vi "Drive Teleop Handler.vi"(10 "Call Context":T1=enum."Stop") -> ()   [LabVIEW 2023]
uses:
  swerve/Type Definitions/Data/Robot Velocities.ctl
  <vilib>/Rock Robotics/WPI/DriverStation/WPI_DriverStationDerivedRobotMode.ctl
  Drive/Implementation/Driving Mode.ctl
  <vilib>/Rock Robotics/WPI/Joystick/XBox Buttons Indexer.ctl
  <vilib>/Rock Robotics/WPI/DriverStation/WPI_DriverStationAllianceInfo.ctl
  ce51abe2-3967-49ec-91df-d4b8ef358bb3.vi
  20f039dc-a6f5-4e97-88ba-31848a91c715.vi
  fdc21bd4-9215-41b8-8367-bf19dde4ba27.vi
  2558f998-dd4e-4154-8f44-6f70b21d0474.vi
  <vilib>/Rock Robotics/WPI/Utilities/WPI_GetSetVariantRefNum.vi
  <vilib>/Rock Robotics/Network Tables/NT Read Number.vi
  <vilib>/Rock Robotics/Network Tables/NT Read Boolean.vi
  Framework/Robot Global Data.vi
  <vilib>/Rock Robotics/Network Tables/NT Write Boolean.vi
panel:
  out "Astra Sees?":bool=TRUE
  out "Li4 Sees?":bool=TRUE
  in  "Red Side":cluster{"Upper lim":dbl, "Lower lim":dbl}={"Upper lim"=12.0, "Lower lim"=6.0}
  in  "Blue Side":cluster{"Upper lim":dbl, "Lower lim":dbl}={"Upper lim"=23.0, "Lower lim"=17.0}
  in  "Deadband Info":T2={"Deadband"=0.05, "Deadband High"=1.0, "Deadband Low"=0.05}
  in  "Max Velocities":T3={"X Velocity"=15.0, "Y Velocity"=15.0, "Rotational \nVelocity"=270.0}
  in  "Sinusoidal Terms":cluster{"Max Velocity":dbl, "Frequency":dbl}
  in  "Teleop Mode":T4(ring)
  in  "Joystick Inputs":T5(array[cluster])
  in  "Send Inputs":bool
  # "reasonable terms"
  # "AprilTag ID bounds"
  # "reasonable terms"
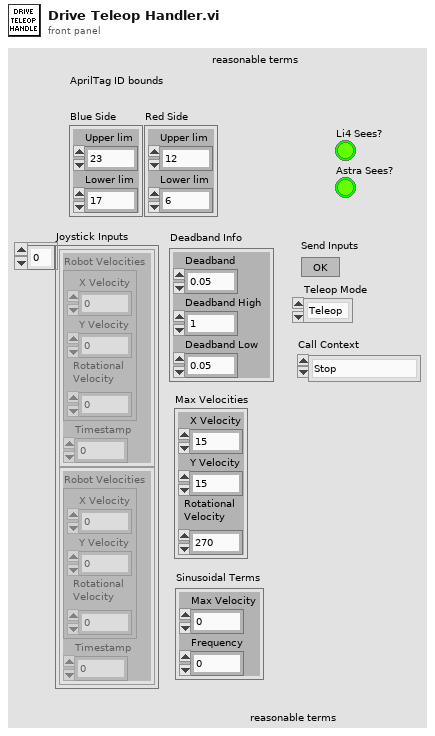
[diagram p1: front panel]
types:
  T1 = typedef "WPI_DriverStationDerivedRobotMode.ctl" = enum16{"Init", "Execute", "Stop"}
  T2 = cluster{"Deadband":dbl, "Deadband High":dbl, "Deadband Low":dbl}
  T3 = typedef "Robot Velocities.ctl" = cluster{"X Velocity":dbl, "Y Velocity":dbl, "Rotational \nVelocity":dbl}
  T4 = enum16{"Teleop", "Simulated Teleop", "Sine Velocity Profiles", "Circle Simulator"}
  T5 = cluster{"Robot Velocities":T3, "Timestamp":dbl}[]
  T6 = typedef "WPI_DriverStationAllianceInfo.ctl" = enum16{"Red", "Blue", "Invalid"}
  T7 = typedef "XBox Buttons Indexer.ctl" = enum16{"A", "B", "X", "Y", "Left Bumper", "Right Bumper", "Back", "Start", "Left Joystick", "Right Joystick"}
  T8 = typedef "Driving Mode.ctl" = enum16{"Robot Centric", "Field Centric"}
  T9 = typedef "WPI_JoystickDevRef.ctl" = cluster{"Device":T10}
  T10 = typedef "WPI_JoystickDeviceEnum.ctl" = enum16{"USB 0", "USB 1", "USB 2", "USB 3", "USB 4", "USB 5"}
  T11 = typedef "CTRE_PigeonIMU_DeviceRef.ctl" = cluster{"DeviceStatus":errorcluster, "Device Number":u8, "Type":T12, "Device ID":u32, "Handle":u64, "UsageFrame":u32, "Library Path":path}
  T12 = typedef "CTRE_PigeonIMU_ConnectionType.ctl" = u32
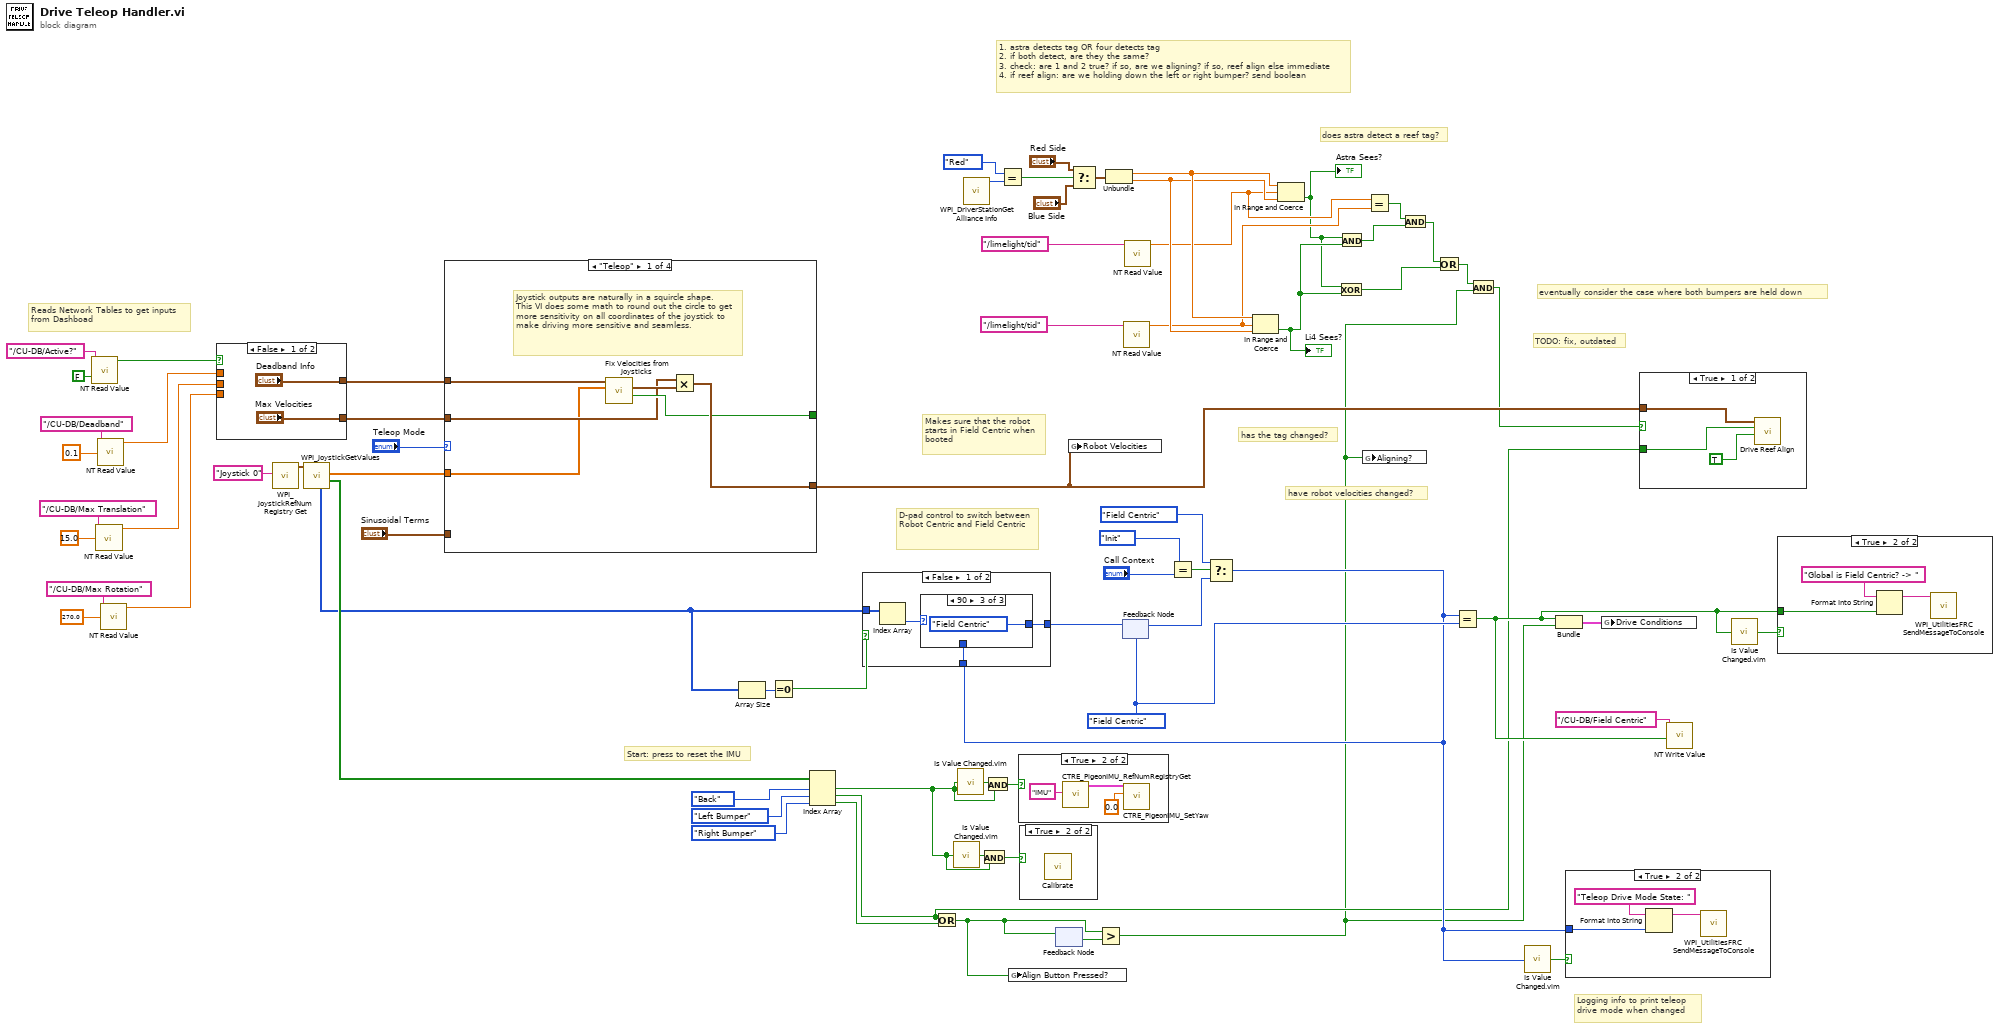
[diagram p0: block diagram]
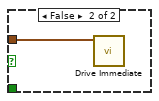
[diagram p2: hidden frame]
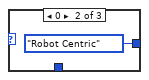
[diagram p8: hidden frame]
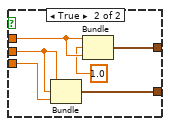
[diagram p10: hidden frame]
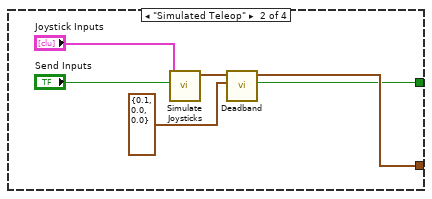
[diagram p11: hidden frame]
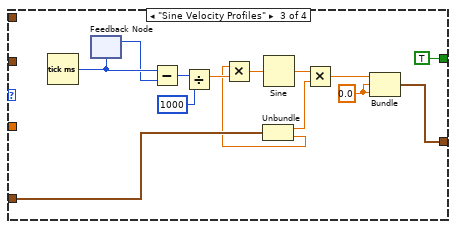
[diagram p12: hidden frame]
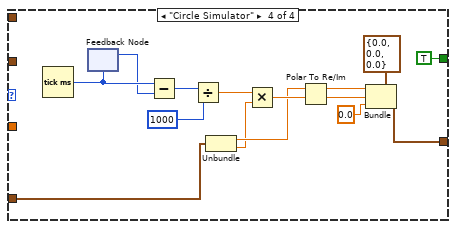
[diagram p13: hidden frame]
diagram:
  w39 = Driving_Mode."Field Centric"
  # "eventually consider the case where both bumpers are held down"
  # "1. astra detects tag OR four detects tag\n2. if both detect, are they the same?\n3. check: are 1 and 2 true? if so, are we aligning? if so, reef align else immediate\n4. if reef align: are we holding down the left or right bumper? send boolean"
  # "have robot velocities changed?"
  # "has the tag changed?"
  # "does astra detect a reef tag?"
  # "TODO: fix, outdated"
  # "Reads Network Tables to get inputs from Dashboad"
  # "Logging info to print teleop drive mode when changed"
  # "Makes sure that the robot starts in Field Centric when booted"
  # "Start: press to reset the IMU"
  # "D-pad control to switch between Robot Centric and Field Centric"
  n1 = call-poly <vilib>:"NT Read Value.vi"("default value"=FALSE ("Default Value"), "name"="/CU-DB/Active?" ("Name")) -> ("value"=w53:bool)  [unwired: 7 in, 2 out]
  n2 = call-poly <vilib>:"NT Read Value.vi"("default value"=15.0 ("Default Value"), "name"="/CU-DB/Max Translation" ("Name")) -> ("value"=w50:dbl)  [unwired: 7 in, 2 out]
  n3 = call-poly <vilib>:"NT Read Value.vi"("default value"=0.1 ("Default Value"), "name"="/CU-DB/Deadband" ("Name")) -> ("value"=w52:dbl)  [unwired: 7 in, 2 out]
  n4 = call-poly <vilib>:"NT Read Value.vi"("default value"=270.0 ("Default Value"), "name"="/CU-DB/Max Rotation" ("Name")) -> ("value"=w49:dbl)  [unwired: 7 in, 2 out]
  n5 = case shown="False" w53 {
    tunnel: w52 -> [_ w78]
    tunnel: ["Deadband Info" w76] -> w51
    tunnel: w50 -> [_ w75]
    tunnel: w49 -> [_ w74]
    tunnel: ["Max Velocities" w73] -> w48
    frame False {
    }
    frame True {
      n6 = Bundle("value"=w75, "value"=w75, "value"=w74) -> (w73:cluster{"value":dbl, "value":dbl, "value":dbl})  [unwired: 1 in]
      n7 = Bundle("value"=w78, "value"=1.0, "value"=w78) -> (w76:cluster{"value":dbl, "value":dbl, "value":dbl})  [unwired: 1 in]
    }
  }
  n8 = call <vilib>:"WPI_JoystickRefNum Registry Get.vi"("refnum name"="Joystick 0") -> ("JoystickDevRef"=w69:T9)  [unwired: 1 in, 9 out]
  n9 = call <vilib>:"WPI_JoystickGetValues.vi"("JoystickDevRef"=w69) -> ("Buttons"=w66:bool[], "Axes"=w68:dbl[], "POVs"=w46:i16[])  [unwired: 6 in, 2 out]
  n10 = case shown="\"Teleop\"" "Teleop Mode" {
    tunnel: w68 -> [w79 _ _ _]
    tunnel: [w84 w90 w95 w117] -> w23
    tunnel: "Sinusoidal Terms" -> [_ _ w94 w107]
    tunnel: w51 -> [w83 _ _ _]
    tunnel: w48 -> [w80 _ _ _]
    tunnel: [w81 w85 TRUE ("Sending Input?") TRUE ("Sending Input?")] -> _
    frame "Teleop" {
      # "Joystick outputs are naturally in a squircle shape.\nThis VI does some math to round out the circle to get more sensitivity on all coordinates of the joystick to make driving more sensitive and seamless."
      n11 = call "Fix Velocities from Joysticks.vi"("Axes"=w79, "Deadband"=w83) -> ("Sending Input?"=w81:bool, "Adjusted Robot Velocities"=w82:T3)  [unwired: 8 in]
      n12 = Multiply(x=w80, y=w82) -> (x*y=w84:T3)
    }
    frame "Simulated Teleop" {
      n13 = call "Simulate Joysticks.vi"("Send Inputs"="Send Inputs", "Joystick Inputs"="Joystick Inputs") -> ("Joystick Inputs"=w87:T3)  [unwired: 9 in]
      n14 = call "Deadband.vi"("Deadband Info"=T2 {"Deadband"=0.1, "Deadband High"=0.0, "Deadband Low"=0.0}, "Robot Velocities"=w87) -> ("Sending Input?"=w85:bool, "Adjusted Robot Velocities"=w90:T3)  [unwired: 8 in]
    }
    frame "Sine Velocity Profiles" {
      w103 = 0.0
      n15 = Tick Count (ms)() -> (millisecond timer value=w97:u32)
      n16 = feedback #1(w97) -> (w96:u32)
      n17 = feedback-in #1(w96) -> ()
      n18 = Subtract(x=w97, y=w96) -> (x-y=w101:u32)
      n19 = Divide(x=w101, y=u32 1000) -> (x/y=w99:dbl)
      n20 = Unbundle(w94) -> ("Max Velocity"=w92:dbl, "Frequency"=w93:dbl)
      n21 = Multiply(x=w93, y=w99) -> (x*y=w98:dbl)
      n22 = Sine(x=w98) -> (sin(x)=w102:dbl)
      n23 = Multiply(x=w102, y=w92) -> (x*y=w104:dbl)
      n24 = Bundle(w104, w103, w103) -> (w95:cluster{dbl, dbl, dbl})  [unwired: 1 in]
    }
    frame "Circle Simulator" {
      n25 = Tick Count (ms)() -> (millisecond timer value=w113:u32)
      n26 = feedback #2(w113) -> (w112:u32)
      n27 = feedback-in #2(w112) -> ()
      n28 = Subtract(x=w113, y=w112) -> (x-y=w115:u32)
      n29 = Divide(x=w115, y=u32 1000) -> (x/y=w109:dbl)
      n30 = Unbundle(w107) -> ("Max Velocity"=w110:dbl, "Frequency"=w108:dbl)
      n31 = Multiply(x=w109, y=w108) -> (x*y=w111:dbl)
      n32 = Polar To Re/Im(2:w111, 3:w110) -> (0:w105:dbl, 1:w106:dbl)
      n33 = Bundle(cluster=T3 {"X Velocity"=0.0, "Y Velocity"=0.0, "Rotational \nVelocity"=0.0} ("Robot Velocities (ft/s and deg/s)"), "X Velocity"=w106, "Y Velocity"=w105, "Rotational \nVelocity"=0.0 ("Rotational \nVelocity")) -> (w117:T3)
    }
  }
  n34 = Array Size(array=w46) -> (size(s)=w45:i32)
  n35 = Equal To 0?(x=w45) -> (x = 0?=w44:bool)
  n36 = Index Array(array=w66, index #1=XBox_Buttons_Indexer."Back" ("XBox Buttons"), index #2=XBox_Buttons_Indexer."Left Bumper" ("XBox Buttons"), index #3=XBox_Buttons_Indexer."Right Bumper" ("XBox Buttons")) -> (element #1=w25:bool, element #2=w26:bool, element #3=w27:bool)
  n37 = Or(x=w26, y=w27) -> (x .or. y?=w1:bool)
  n38 = call "Is Value Changed.vim"("value"=w25) -> ("changed or first call?"=w33:bool)
  n39 = call "Is Value Changed.vim"("value"=w25) -> ("changed or first call?"=w65:bool)
  n40 = call <vilib>:"WPI_DriverStationGet Alliance Info.vi"() -> ("Alliance"=w20:T6)  [unwired: 6 in, 5 out]
  n41 = And(x=w33, y=w25) -> (x .and. y?=w32:bool)
  n42 = And(x=w65, y=w25) -> (x .and. y?=w64:bool)
  n43 = Equal?(x=WPI_DriverStationAllianceInfo."Red", y=w20) -> (x = y?=w18:bool)
  n44 = global write "Robot Global Data.vi" "Align Button Pressed?"(w1) -> ()
  n45 = case shown="True" w64 {
    frame False {
    }
    frame True {
      n46 = call <vilib>:"CTRE_PigeonIMU_RefNumRegistryGet.vi"("refnum name"="IMU") -> ("PigeonIMUDevRef"=w121:T11)  [unwired: 9 in, 1 out]
      n47 = call <vilib>:"CTRE_PigeonIMU_SetYaw.vi"("Value"=0.0, "PigeonIMUDevRef"=w121) -> ()  [unwired: 8 in, 2 out]
    }
  }
  n48 = case shown="True" w32 {
    frame False {
    }
    frame True {
      n49 = call "Calibrate.vi"() -> ()  [unwired: 11 in, 1 out]
    }
  }
  n50 = feedback-in #3(w1) -> ()
  n51 = feedback #3() -> (w5:bool)  [unwired: 1 in]
  n52 = global write "Robot Global Data.vi" "Robot Velocities"(w23) -> ()
  n53 = Select(t="Red Side", s=w18, f="Blue Side") -> (s? t:f=w22:cluster{"Upper lim":dbl, "Lower lim":dbl})
  n54 = Greater?(x=w1, y=w5) -> (0:w4:bool)
  n55 = Unbundle(w22) -> ("Upper lim"=w15:dbl, "Lower lim"=w14:dbl)
  n56 = feedback #4(w39) -> (w38:T8)
  n57 = call-poly <vilib>:"NT Read Value.vi"("name"="/limelight/tid") -> ("value"=w12:dbl)  [unwired: 8 in, 2 out]
  n58 = call-poly <vilib>:"NT Read Value.vi"("name"="/limelight/tid") -> ("value"=w13:dbl)  [unwired: 8 in, 2 out]
  n59 = Equal?(x=WPI_DriverStationDerivedRobotMode."Init" ("y"), y="Call Context") -> (x = y?=w41:bool)
  n60 = Select(t=Driving_Mode."Field Centric" ("x"), s=w41, f=w38) -> (s? t:f=w35:T8)
  n61 = case shown="False" w44 {
    tunnel: [w125 w130] -> w67
    tunnel: w35 -> [w124 w130]
    tunnel: w46 -> [w123 _]
    frame False {
      n62 = Index Array(array=w123) -> (element=w126:i16)  [unwired: 1 in]
      n63 = case shown="90" w126 {
        tunnel: [w127 Driving_Mode."Robot Centric" Driving_Mode."Field Centric"] -> w125
        tunnel: w124 -> [w127 _ _]
        frame -1, Default {
        }
        frame 0 {
        }
        frame 90 {
        }
      }
    }
    frame True {
    }
  }
  n64 = feedback-in #4(w67) -> ()
  n65 = In Range and Coerce(upper limit=w15, x=w12, lower limit=w14) -> (In Range?=w3:bool)  [unwired: 1 out]
  "Li4 Sees?" <- w3
  n66 = In Range and Coerce(upper limit=w15, x=w13, lower limit=w14) -> (In Range?=w2:bool)  [unwired: 1 out]
  "Astra Sees?" <- w2
  n67 = Exclusive Or(1:w3, 2:w2) -> (0:w8:bool)
  n68 = And(x=w2, y=w3) -> (x .and. y?=w10:bool)
  n69 = global write "Robot Global Data.vi" "Aligning?"(w4) -> ()
  n70 = Equal?(x=w13, y=w12) -> (x = y?=w11:bool)
  n71 = And(x=w11, y=w10) -> (x .and. y?=w9:bool)
  n72 = Or(x=w9, y=w8) -> (x .or. y?=w7:bool)
  n73 = Equal?(x=w35, y=w39) -> (x = y?=w36:bool)
  n74 = And(x=w7, y=w4) -> (x .and. y?=w6:bool)
  n75 = call "Is Value Changed.vim"("value"=w35) -> ("changed or first call?"=w34:bool)
  n76 = Bundle(w36, w4) -> (w28:cluster{bool, bool})  [unwired: 1 in]
  n77 = case shown="True" w34 {
    tunnel: w35 -> [_ w131]
    frame False {
    }
    frame True {
      n78 = Format Into String(initial string="Teleop Drive Mode State: ", w131) -> (resulting string=w133:string)  [unwired: 2 in, 1 out]
      n79 = call <vilib>:"WPI_UtilitiesFRC SendMessageToConsole.vi"("Message"=w133) -> ()  [unwired: 14 in, 1 out]
    }
  }
  n80 = global write "Robot Global Data.vi" "Drive Conditions"(w28) -> ()
  n81 = case shown="True" w6 {
    tunnel: w23 -> [w135 w137]
    tunnel: w26 -> [w136 _]
    frame True {
      n82 = call "Drive Reef Align.vi"("Angle Align"=TRUE, "Left Side?"=w136, "Robot Velocities"=w135) -> ()  [unwired: 8 in, 1 out]
    }
    frame False {
      n83 = call "Drive Immediate.vi"("Robot Velocities"=w137) -> ()  [unwired: 10 in, 1 out]
    }
  }
  n84 = call-poly <vilib>:"NT Write Value.vi"("value"=w36, "name"="/CU-DB/Field Centric") -> ()  [unwired: 9 in, 1 out]
  n85 = call "Is Value Changed.vim"("value"=w36) -> ("changed or first call?"=w37:bool)
  n86 = case shown="True" w37 {
    tunnel: w36 -> [_ w139]
    frame False {
    }
    frame True {
      n87 = Format Into String(initial string="Global is Field Centric? -> ", w139) -> (resulting string=w140:string)  [unwired: 2 in, 1 out]
      n88 = call <vilib>:"WPI_UtilitiesFRC SendMessageToConsole.vi"("Message"=w140) -> ()  [unwired: 14 in, 1 out]
    }
  }
